vi "SplitInputsTo64PinArrays.vi"(11 "Inputs":T2[](array[typedef])) -> (0 "Pads 49-64":T1(array[cluster]), 1 "Pads 33-48":T1(array[cluster]), 2 "Pads 17-32":T1(array[cluster]), 3 "Pads 1-16":T1(array[cluster]))   [LabVIEW 2012, in "Virtual-PGA.lvlib"]
uses:
  Virtual-PGA.lvlib
  Public/Controls/Input.ctl
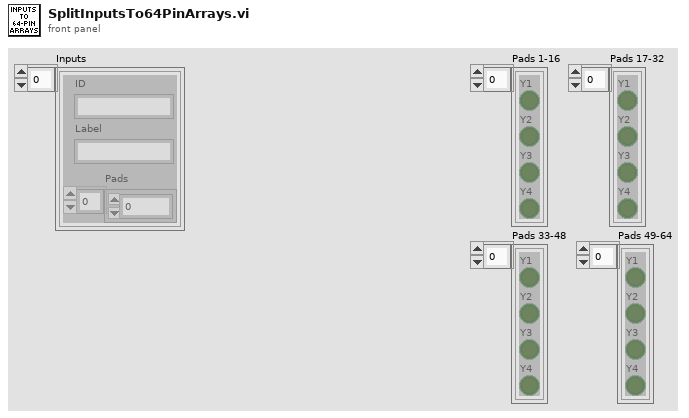
[diagram p1: front panel]
types:
  T1 = cluster{"Y1":bool, "Y2":bool, "Y3":bool, "Y4":bool}[]
  T2 = typedef "Virtual-PGA.lvlib/Input.ctl" = cluster{"ID":string, "Label":string, "Pads":u32[]}
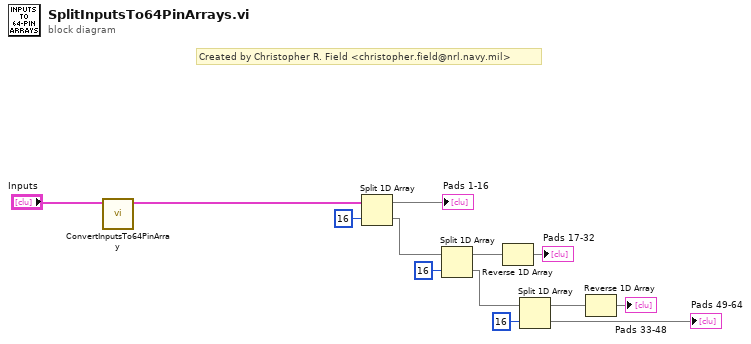
[diagram p0: block diagram]
diagram:
  # "Created by Christopher R. Field <christopher.field@nrl.navy.mil>"
  n1 = call "ConvertInputsTo64PinArray.vi"("Inputs"="Inputs") -> ("64-Pin Array"=w1:T1)  [unwired: 10 in]
  n2 = Split 1D Array(array=w1, index=16) -> (first subarray=→"Pads 1-16":T1, second subarray=w10:T1)
  n3 = Split 1D Array(array=w10, index=16) -> (first subarray=w7:T1, second subarray=w9:T1)
  n4 = Reverse 1D Array(array=w7) -> (reversed array=→"Pads 17-32":T1)
  n5 = Split 1D Array(array=w9, index=16) -> (first subarray=w5:T1, second subarray=→"Pads 49-64":T1)
  n6 = Reverse 1D Array(array=w5) -> (reversed array=→"Pads 33-48":T1)
